vi "RTS Wago Data 4.vi"(8 "Error In":errorcluster, 10 "Station":u8, 11 "Chamber 1 Data in":T1 {"Room PID Settings"."Room Dehumid Temperature I (*RM Dehum I1)" max=30000 step=1; "Room PID Settings"."Room Dehumid Temperature P (*RM Dehum P1)" max=30000 step=1; "Room PID Settings"."Room Cool Temperature I (*RM Cool I1)" max=30000 step=1; "Room PID Settings"."Room Cool Temperature P (*RM Cool P1)" max=30000 step=1; "Room PID Settings"."Room Heat I (*RM Heat I1)" max=30000 step=1; "Room PID Settings"."Room Heat P (*RM Heat P1)" max=30000 step=1; "Room PID Settings"."Room Humidity I (*RM Hum I1)" max=30000 step=1; "Room PID Settings"."Room Humidity P (*RM Hum P1)" max=30000 step=1; "Room PID Settings"."Room Dry I (*RM Dry I1)" max=30000 step=1; "Room PID Settings"."Room Dry P(*RM Dry P1)" max=30000 step=1; "Station 8"."Voltage (V):Element 1 Avg" format="%.3g"; "Station 8"."Voltage (V):Element 2 Avg" format="%.3g"; "Station 8"."Max Watt Hours" format="%.3g"; "Station 8"."Power Factor:Element 2" format="%.3g"; "Station 8"."Power Factor:Element 1" format="%.3g"; "Station 8"."Apparent Power (VA):Element 2" format="%.3g"; "Station 8"."Apparent Power (VA):Element 1" format="%.3g"; "Station 8"."Frequency (Hz):Element 1" format="%.3g"; "Station 8"."Time:Element 1" format="%.3g"; "Station 8"."Voltage Crest Factor:Element 2" format="%.3g"; "Station 8"."Voltage Crest Factor:Element 1" format="%.3g"; "Station 8"."Voltage Harmonic (%):Element 2" format="%.3g"; "Station 8"."Voltage Harmonic (%):Element 1" format="%.3g"; "Station 8"."Current Crest Factor:Element 2" format="%.3g"; "Station 8"."Current Crest Factor:Element 1" format="%.3g"; "Station 8"."Voltage (V):Element 1" format="%.3g"; "Station 8"."Voltage (V):Element 2" format="%.3g"; "Station 8"."Watt Hours (Wh):Sigma" format="%.3f"; "Station 8"."Power (W):Sigma" format="%.3g"; "Station 8"."Current (A):Element 2" format="%.3g"; "Station 8"."Current (A):Element 1" format="%.3g"; "Station 7"."Voltage (V):Element 1 Avg" format="%.3g"; "Station 7"."Voltage (V):Element 2 Avg" format="%.3g"; "Station 7"."Max Watt Hours" format="%.3g"; "Station 7"."Power Factor:Element 2" format="%.3g"; "Station 7"."Power Factor:Element 1" format="%.3g"; "Station 7"."Apparent Power (VA):Element 2" format="%.3g"; "Station 7"."Apparent Power (VA):Element 1" format="%.3g"; "Station 7"."Frequency (Hz):Element 1" format="%.3g"; "Station 7"."Time:Element 1" format="%.3g"; "Station 7"."Voltage Crest Factor:Element 2" format="%.3g"; "Station 7"."Voltage Crest Factor:Element 1" format="%.3g"; "Station 7"."Voltage Harmonic (%):Element 2" format="%.3g"; "Station 7"."Voltage Harmonic (%):Element 1" format="%.3g"; "Station 7"."Current Crest Factor:Element 2" format="%.3g"; "Station 7"."Current Crest Factor:Element 1" format="%.3g"; "Station 7"."Voltage (V):Element 1" format="%.3g"; "Station 7"."Voltage (V):Element 2" format="%.3g"; "Station 7"."Watt Hours (Wh):Sigma" format="%.3f"; "Station 7"."Power (W):Sigma" format="%.3g"; "Station 7"."Current (A):Element 2" format="%.3g"; "Station 7"."Current (A):Element 1" format="%.3g"; "Station 6"."Voltage (V):Element 1 Avg" format="%.3g"; "Station 6"."Voltage (V):Element 2 Avg" format="%.3g"; "Station 6"."Max Watt Hours" format="%.3g"; "Station 6"."Power Factor:Element 2" format="%.3g"; "Station 6"."Power Factor:Element 1" format="%.3g"; "Station 6"."Apparent Power (VA):Element 2" format="%.3g"; "Station 6"."Apparent Power (VA):Element 1" format="%.3g"; "Station 6"."Frequency (Hz):Element 1" format="%.3g"; "Station 6"."Time:Element 1" format="%.3g"; "Station 6"."Voltage Crest Factor:Element 2" format="%.3g"; "Station 6"."Voltage Crest Factor:Element 1" format="%.3g"; "Station 6"."Voltage Harmonic (%):Element 2" format="%.3g"; "Station 6"."Voltage Harmonic (%):Element 1" format="%.3g"; "Station 6"."Current Crest Factor:Element 2" format="%.3g"; "Station 6"."Current Crest Factor:Element 1" format="%.3g"; "Station 6"."Voltage (V):Element 1" format="%.3g"; "Station 6"."Voltage (V):Element 2" format="%.3g"; "Station 6"."Watt Hours (Wh):Sigma" format="%.3f"; "Station 6"."Power (W):Sigma" format="%.3g"; "Station 6"."Current (A):Element 2" format="%.3g"; "Station 6"."Current (A):Element 1" format="%.3g"; "Station 5"."Voltage (V):Element 1 Avg" format="%.3g"; "Station 5"."Voltage (V):Element 2 Avg" format="%.3g"; "Station 5"."Max Watt Hours" format="%.3g"; "Station 5"."Power Factor:Element 2" format="%.3g"; "Station 5"."Power Factor:Element 1" format="%.3g"; "Station 5"."Apparent Power (VA):Element 2" format="%.3g"; "Station 5"."Apparent Power (VA):Element 1" format="%.3g"; "Station 5"."Frequency (Hz):Element 1" format="%.3g"; "Station 5"."Time:Element 1" format="%.3g"; "Station 5"."Voltage Crest Factor:Element 2" format="%.3g"; "Station 5"."Voltage Crest Factor:Element 1" format="%.3g"; "Station 5"."Voltage Harmonic (%):Element 2" format="%.3g"; "Station 5"."Voltage Harmonic (%):Element 1" format="%.3g"; "Station 5"."Current Crest Factor:Element 2" format="%.3g"; "Station 5"."Current Crest Factor:Element 1" format="%.3g"; "Station 5"."Voltage (V):Element 1" format="%.3g"; "Station 5"."Voltage (V):Element 2" format="%.3g"; "Station 5"."Watt Hours (Wh):Sigma" format="%.3f"; "Station 5"."Power (W):Sigma" format="%.3g"; "Station 5"."Current (A):Element 2" format="%.3g"; "Station 5"."Current (A):Element 1" format="%.3g"; "Station 4"."Voltage (V):Element 1 Avg" format="%.3g"; "Station 4"."Voltage (V):Element 2 Avg" format="%.3g"; "Station 4"."Max Watt Hours" format="%.3g"; "Station 4"."Power Factor:Element 2" format="%.3g"; "Station 4"."Power Factor:Element 1" format="%.3g"; "Station 4"."Apparent Power (VA):Element 2" format="%.3g"; "Station 4"."Apparent Power (VA):Element 1" format="%.3g"; "Station 4"."Frequency (Hz):Element 1" format="%.3g"; "Station 4"."Time:Element 1" format="%.3g"; "Station 4"."Voltage Crest Factor:Element 2" format="%.3g"; "Station 4"."Voltage Crest Factor:Element 1" format="%.3g"; "Station 4"."Voltage Harmonic (%):Element 2" format="%.3g"; "Station 4"."Voltage Harmonic (%):Element 1" format="%.3g"; "Station 4"."Current Crest Factor:Element 2" format="%.3g"; "Station 4"."Current Crest Factor:Element 1" format="%.3g"; "Station 4"."Voltage (V):Element 1" format="%.3g"; "Station 4"."Voltage (V):Element 2" format="%.3g"; "Station 4"."Watt Hours (Wh):Sigma" format="%.3f"; "Station 4"."Power (W):Sigma" format="%.3g"; "Station 4"."Current (A):Element 2" format="%.3g"; "Station 4"."Current (A):Element 1" format="%.3g"; "Station 3"."Voltage (V):Element 1 Avg" format="%.3g"; "Station 3"."Voltage (V):Element 2 Avg" format="%.3g"; "Station 3"."Max Watt Hours" format="%.3g"; "Station 3"."Power Factor:Element 2" format="%.3g"; "Station 3"."Power Factor:Element 1" format="%.3g"; "Station 3"."Apparent Power (VA):Element 2" format="%.3g"; "Station 3"."Apparent Power (VA):Element 1" format="%.3g"; "Station 3"."Frequency (Hz):Element 1" format="%.3g"; "Station 3"."Time:Element 1" format="%.3g"; "Station 3"."Voltage Crest Factor:Element 2" format="%.3g"; "Station 3"."Voltage Crest Factor:Element 1" format="%.3g"; "Station 3"."Voltage Harmonic (%):Element 2" format="%.3g"; "Station 3"."Voltage Harmonic (%):Element 1" format="%.3g"; "Station 3"."Current Crest Factor:Element 2" format="%.3g"; "Station 3"."Current Crest Factor:Element 1" format="%.3g"; "Station 3"."Voltage (V):Element 1" format="%.3g"; "Station 3"."Voltage (V):Element 2" format="%.3g"; "Station 3"."Watt Hours (Wh):Sigma" format="%.3f"; "Station 3"."Power (W):Sigma" format="%.3g"; "Station 3"."Current (A):Element 2" format="%.3g"; "Station 3"."Current (A):Element 1" format="%.3g"; "Station 2"."Voltage (V):Element 1 Avg" format="%.3g"; "Station 2"."Voltage (V):Element 2 Avg" format="%.3g"; "Station 2"."Max Watt Hours" format="%.3g"; "Station 2"."Power Factor:Element 2" format="%.3g"; "Station 2"."Power Factor:Element 1" format="%.3g"; "Station 2"."Apparent Power (VA):Element 2" format="%.3g"; "Station 2"."Apparent Power (VA):Element 1" format="%.3g"; "Station 2"."Frequency (Hz):Element 1" format="%.3g"; "Station 2"."Time:Element 1" format="%.3g"; "Station 2"."Voltage Crest Factor:Element 2" format="%.3g"; "Station 2"."Voltage Crest Factor:Element 1" format="%.3g"; "Station 2"."Voltage Harmonic (%):Element 2" format="%.3g"; "Station 2"."Voltage Harmonic (%):Element 1" format="%.3g"; "Station 2"."Current Crest Factor:Element 2" format="%.3g"; "Station 2"."Current Crest Factor:Element 1" format="%.3g"; "Station 2"."Voltage (V):Element 1" format="%.3g"; "Station 2"."Voltage (V):Element 2" format="%.3g"; "Station 2"."Watt Hours (Wh):Sigma" format="%.3f"; "Station 2"."Power (W):Sigma" format="%.3g"; "Station 2"."Current (A):Element 2" format="%.3g"; "Station 2"."Current (A):Element 1" format="%.3g"; "Station 1"."Voltage (V):Element 1 Avg" format="%.3g"; "Station 1"."Voltage (V):Element 2 Avg" format="%.3g"; "Station 1"."Max Watt Hours" format="%.3g"; "Station 1"."Power Factor:Element 2" format="%.3g"; "Station 1"."Power Factor:Element 1" format="%.3g"; "Station 1"."Apparent Power (VA):Element 2" format="%.3g"; "Station 1"."Apparent Power (VA):Element 1" format="%.3g"; "Station 1"."Frequency (Hz):Element 1" format="%.3g"; "Station 1"."Time:Element 1" format="%.3g"; "Station 1"."Voltage Crest Factor:Element 2" format="%.3g"; "Station 1"."Voltage Crest Factor:Element 1" format="%.3g"; "Station 1"."Voltage Harmonic (%):Element 2" format="%.3g"; "Station 1"."Voltage Harmonic (%):Element 1" format="%.3g"; "Station 1"."Current Crest Factor:Element 2" format="%.3g"; "Station 1"."Current Crest Factor:Element 1" format="%.3g"; "Station 1"."Voltage (V):Element 1" format="%.3g"; "Station 1"."Voltage (V):Element 2" format="%.3g"; "Station 1"."Watt Hours (Wh):Sigma" format="%.3f"; "Station 1"."Power (W):Sigma" format="%.3g"; "Station 1"."Current (A):Element 2" format="%.3g"; "Station 1"."Current (A):Element 1" format="%.3g"}) -> (0 "Error Out":errorcluster, 1 "Data 4 (DBL)":dbl[](array[numeric]), 2 "Data 4":string[][](array[string]), 3 "Chamber 1 Data Out":T1 {"Room PID Settings"."Room Dehumid Temperature I (*RM Dehum I1)" max=30000 step=1; "Room PID Settings"."Room Dehumid Temperature P (*RM Dehum P1)" max=30000 step=1; "Room PID Settings"."Room Cool Temperature I (*RM Cool I1)" max=30000 step=1; "Room PID Settings"."Room Cool Temperature P (*RM Cool P1)" max=30000 step=1; "Room PID Settings"."Room Heat I (*RM Heat I1)" max=30000 step=1; "Room PID Settings"."Room Heat P (*RM Heat P1)" max=30000 step=1; "Room PID Settings"."Room Humidity I (*RM Hum I1)" max=30000 step=1; "Room PID Settings"."Room Humidity P (*RM Hum P1)" max=30000 step=1; "Room PID Settings"."Room Dry I (*RM Dry I1)" max=30000 step=1; "Room PID Settings"."Room Dry P(*RM Dry P1)" max=30000 step=1; "Station 8"."Voltage (V):Element 1 Avg" format="%.3g"; "Station 8"."Voltage (V):Element 2 Avg" format="%.3g"; "Station 8"."Max Watt Hours" format="%.3g"; "Station 8"."Power Factor:Element 2" format="%.3g"; "Station 8"."Power Factor:Element 1" format="%.3g"; "Station 8"."Apparent Power (VA):Element 2" format="%.3g"; "Station 8"."Apparent Power (VA):Element 1" format="%.3g"; "Station 8"."Frequency (Hz):Element 1" format="%.3g"; "Station 8"."Time:Element 1" format="%.3g"; "Station 8"."Voltage Crest Factor:Element 2" format="%.3g"; "Station 8"."Voltage Crest Factor:Element 1" format="%.3g"; "Station 8"."Voltage Harmonic (%):Element 2" format="%.3g"; "Station 8"."Voltage Harmonic (%):Element 1" format="%.3g"; "Station 8"."Current Crest Factor:Element 2" format="%.3g"; "Station 8"."Current Crest Factor:Element 1" format="%.3g"; "Station 8"."Voltage (V):Element 1" format="%.3g"; "Station 8"."Voltage (V):Element 2" format="%.3g"; "Station 8"."Watt Hours (Wh):Sigma" format="%.3f"; "Station 8"."Power (W):Sigma" format="%.3g"; "Station 8"."Current (A):Element 2" format="%.3g"; "Station 8"."Current (A):Element 1" format="%.3g"; "Station 7"."Voltage (V):Element 1 Avg" format="%.3g"; "Station 7"."Voltage (V):Element 2 Avg" format="%.3g"; "Station 7"."Max Watt Hours" format="%.3g"; "Station 7"."Power Factor:Element 2" format="%.3g"; "Station 7"."Power Factor:Element 1" format="%.3g"; "Station 7"."Apparent Power (VA):Element 2" format="%.3g"; "Station 7"."Apparent Power (VA):Element 1" format="%.3g"; "Station 7"."Frequency (Hz):Element 1" format="%.3g"; "Station 7"."Time:Element 1" format="%.3g"; "Station 7"."Voltage Crest Factor:Element 2" format="%.3g"; "Station 7"."Voltage Crest Factor:Element 1" format="%.3g"; "Station 7"."Voltage Harmonic (%):Element 2" format="%.3g"; "Station 7"."Voltage Harmonic (%):Element 1" format="%.3g"; "Station 7"."Current Crest Factor:Element 2" format="%.3g"; "Station 7"."Current Crest Factor:Element 1" format="%.3g"; "Station 7"."Voltage (V):Element 1" format="%.3g"; "Station 7"."Voltage (V):Element 2" format="%.3g"; "Station 7"."Watt Hours (Wh):Sigma" format="%.3f"; "Station 7"."Power (W):Sigma" format="%.3g"; "Station 7"."Current (A):Element 2" format="%.3g"; "Station 7"."Current (A):Element 1" format="%.3g"; "Station 6"."Voltage (V):Element 1 Avg" format="%.3g"; "Station 6"."Voltage (V):Element 2 Avg" format="%.3g"; "Station 6"."Max Watt Hours" format="%.3g"; "Station 6"."Power Factor:Element 2" format="%.3g"; "Station 6"."Power Factor:Element 1" format="%.3g"; "Station 6"."Apparent Power (VA):Element 2" format="%.3g"; "Station 6"."Apparent Power (VA):Element 1" format="%.3g"; "Station 6"."Frequency (Hz):Element 1" format="%.3g"; "Station 6"."Time:Element 1" format="%.3g"; "Station 6"."Voltage Crest Factor:Element 2" format="%.3g"; "Station 6"."Voltage Crest Factor:Element 1" format="%.3g"; "Station 6"."Voltage Harmonic (%):Element 2" format="%.3g"; "Station 6"."Voltage Harmonic (%):Element 1" format="%.3g"; "Station 6"."Current Crest Factor:Element 2" format="%.3g"; "Station 6"."Current Crest Factor:Element 1" format="%.3g"; "Station 6"."Voltage (V):Element 1" format="%.3g"; "Station 6"."Voltage (V):Element 2" format="%.3g"; "Station 6"."Watt Hours (Wh):Sigma" format="%.3f"; "Station 6"."Power (W):Sigma" format="%.3g"; "Station 6"."Current (A):Element 2" format="%.3g"; "Station 6"."Current (A):Element 1" format="%.3g"; "Station 5"."Voltage (V):Element 1 Avg" format="%.3g"; "Station 5"."Voltage (V):Element 2 Avg" format="%.3g"; "Station 5"."Max Watt Hours" format="%.3g"; "Station 5"."Power Factor:Element 2" format="%.3g"; "Station 5"."Power Factor:Element 1" format="%.3g"; "Station 5"."Apparent Power (VA):Element 2" format="%.3g"; "Station 5"."Apparent Power (VA):Element 1" format="%.3g"; "Station 5"."Frequency (Hz):Element 1" format="%.3g"; "Station 5"."Time:Element 1" format="%.3g"; "Station 5"."Voltage Crest Factor:Element 2" format="%.3g"; "Station 5"."Voltage Crest Factor:Element 1" format="%.3g"; "Station 5"."Voltage Harmonic (%):Element 2" format="%.3g"; "Station 5"."Voltage Harmonic (%):Element 1" format="%.3g"; "Station 5"."Current Crest Factor:Element 2" format="%.3g"; "Station 5"."Current Crest Factor:Element 1" format="%.3g"; "Station 5"."Voltage (V):Element 1" format="%.3g"; "Station 5"."Voltage (V):Element 2" format="%.3g"; "Station 5"."Watt Hours (Wh):Sigma" format="%.3f"; "Station 5"."Power (W):Sigma" format="%.3g"; "Station 5"."Current (A):Element 2" format="%.3g"; "Station 5"."Current (A):Element 1" format="%.3g"; "Station 4"."Voltage (V):Element 1 Avg" format="%.3g"; "Station 4"."Voltage (V):Element 2 Avg" format="%.3g"; "Station 4"."Max Watt Hours" format="%.3g"; "Station 4"."Power Factor:Element 2" format="%.3g"; "Station 4"."Power Factor:Element 1" format="%.3g"; "Station 4"."Apparent Power (VA):Element 2" format="%.3g"; "Station 4"."Apparent Power (VA):Element 1" format="%.3g"; "Station 4"."Frequency (Hz):Element 1" format="%.3g"; "Station 4"."Time:Element 1" format="%.3g"; "Station 4"."Voltage Crest Factor:Element 2" format="%.3g"; "Station 4"."Voltage Crest Factor:Element 1" format="%.3g"; "Station 4"."Voltage Harmonic (%):Element 2" format="%.3g"; "Station 4"."Voltage Harmonic (%):Element 1" format="%.3g"; "Station 4"."Current Crest Factor:Element 2" format="%.3g"; "Station 4"."Current Crest Factor:Element 1" format="%.3g"; "Station 4"."Voltage (V):Element 1" format="%.3g"; "Station 4"."Voltage (V):Element 2" format="%.3g"; "Station 4"."Watt Hours (Wh):Sigma" format="%.3f"; "Station 4"."Power (W):Sigma" format="%.3g"; "Station 4"."Current (A):Element 2" format="%.3g"; "Station 4"."Current (A):Element 1" format="%.3g"; "Station 3"."Voltage (V):Element 1 Avg" format="%.3g"; "Station 3"."Voltage (V):Element 2 Avg" format="%.3g"; "Station 3"."Max Watt Hours" format="%.3g"; "Station 3"."Power Factor:Element 2" format="%.3g"; "Station 3"."Power Factor:Element 1" format="%.3g"; "Station 3"."Apparent Power (VA):Element 2" format="%.3g"; "Station 3"."Apparent Power (VA):Element 1" format="%.3g"; "Station 3"."Frequency (Hz):Element 1" format="%.3g"; "Station 3"."Time:Element 1" format="%.3g"; "Station 3"."Voltage Crest Factor:Element 2" format="%.3g"; "Station 3"."Voltage Crest Factor:Element 1" format="%.3g"; "Station 3"."Voltage Harmonic (%):Element 2" format="%.3g"; "Station 3"."Voltage Harmonic (%):Element 1" format="%.3g"; "Station 3"."Current Crest Factor:Element 2" format="%.3g"; "Station 3"."Current Crest Factor:Element 1" format="%.3g"; "Station 3"."Voltage (V):Element 1" format="%.3g"; "Station 3"."Voltage (V):Element 2" format="%.3g"; "Station 3"."Watt Hours (Wh):Sigma" format="%.3f"; "Station 3"."Power (W):Sigma" format="%.3g"; "Station 3"."Current (A):Element 2" format="%.3g"; "Station 3"."Current (A):Element 1" format="%.3g"; "Station 2"."Voltage (V):Element 1 Avg" format="%.3g"; "Station 2"."Voltage (V):Element 2 Avg" format="%.3g"; "Station 2"."Max Watt Hours" format="%.3g"; "Station 2"."Power Factor:Element 2" format="%.3g"; "Station 2"."Power Factor:Element 1" format="%.3g"; "Station 2"."Apparent Power (VA):Element 2" format="%.3g"; "Station 2"."Apparent Power (VA):Element 1" format="%.3g"; "Station 2"."Frequency (Hz):Element 1" format="%.3g"; "Station 2"."Time:Element 1" format="%.3g"; "Station 2"."Voltage Crest Factor:Element 2" format="%.3g"; "Station 2"."Voltage Crest Factor:Element 1" format="%.3g"; "Station 2"."Voltage Harmonic (%):Element 2" format="%.3g"; "Station 2"."Voltage Harmonic (%):Element 1" format="%.3g"; "Station 2"."Current Crest Factor:Element 2" format="%.3g"; "Station 2"."Current Crest Factor:Element 1" format="%.3g"; "Station 2"."Voltage (V):Element 1" format="%.3g"; "Station 2"."Voltage (V):Element 2" format="%.3g"; "Station 2"."Watt Hours (Wh):Sigma" format="%.3f"; "Station 2"."Power (W):Sigma" format="%.3g"; "Station 2"."Current (A):Element 2" format="%.3g"; "Station 2"."Current (A):Element 1" format="%.3g"; "Station 1"."Voltage (V):Element 1 Avg" format="%.3g"; "Station 1"."Voltage (V):Element 2 Avg" format="%.3g"; "Station 1"."Max Watt Hours" format="%.3g"; "Station 1"."Power Factor:Element 2" format="%.3g"; "Station 1"."Power Factor:Element 1" format="%.3g"; "Station 1"."Apparent Power (VA):Element 2" format="%.3g"; "Station 1"."Apparent Power (VA):Element 1" format="%.3g"; "Station 1"."Frequency (Hz):Element 1" format="%.3g"; "Station 1"."Time:Element 1" format="%.3g"; "Station 1"."Voltage Crest Factor:Element 2" format="%.3g"; "Station 1"."Voltage Crest Factor:Element 1" format="%.3g"; "Station 1"."Voltage Harmonic (%):Element 2" format="%.3g"; "Station 1"."Voltage Harmonic (%):Element 1" format="%.3g"; "Station 1"."Current Crest Factor:Element 2" format="%.3g"; "Station 1"."Current Crest Factor:Element 1" format="%.3g"; "Station 1"."Voltage (V):Element 1" format="%.3g"; "Station 1"."Voltage (V):Element 2" format="%.3g"; "Station 1"."Watt Hours (Wh):Sigma" format="%.3f"; "Station 1"."Power (W):Sigma" format="%.3g"; "Station 1"."Current (A):Element 2" format="%.3g"; "Station 1"."Current (A):Element 1" format="%.3g"})   [LabVIEW 2016]
uses:
  Type Definitions/RTS Chamber Data.ctl
  Utility/Type Definitions/UTILITY Power Data.ctl
  Type Definitions/RTS Chamber TCs.ctl
  Type Definitions/RTS MX5 AUX Data.ctl
  Drivers/WAGO 750-881/Type Definitions/Wago Door Relays.ctl
  Drivers/WAGO 750-881/Type Definitions/Wago Contactor Settings.ctl
  Drivers/WAGO 750-881/Type Definitions/Wago Ground Leakage.ctl
  Drivers/WAGO 750-881/Type Definitions/Wago Measured Input Data.ctl
  Drivers/WAGO 750-881/Type Definitions/Wago Room Setpoint Targets.ctl
  Drivers/WAGO 750-881/Type Definitions/Wago Room PID Settings.ctl
  Drivers/WAGO 750-881/Type Definitions/Wago Room Condtions.ctl
panel:
  # "APLUS"
  # "MX100"
  # "Wago Controller"
  # "APLUS"
  # "MX100"
  # "Wago Controller"
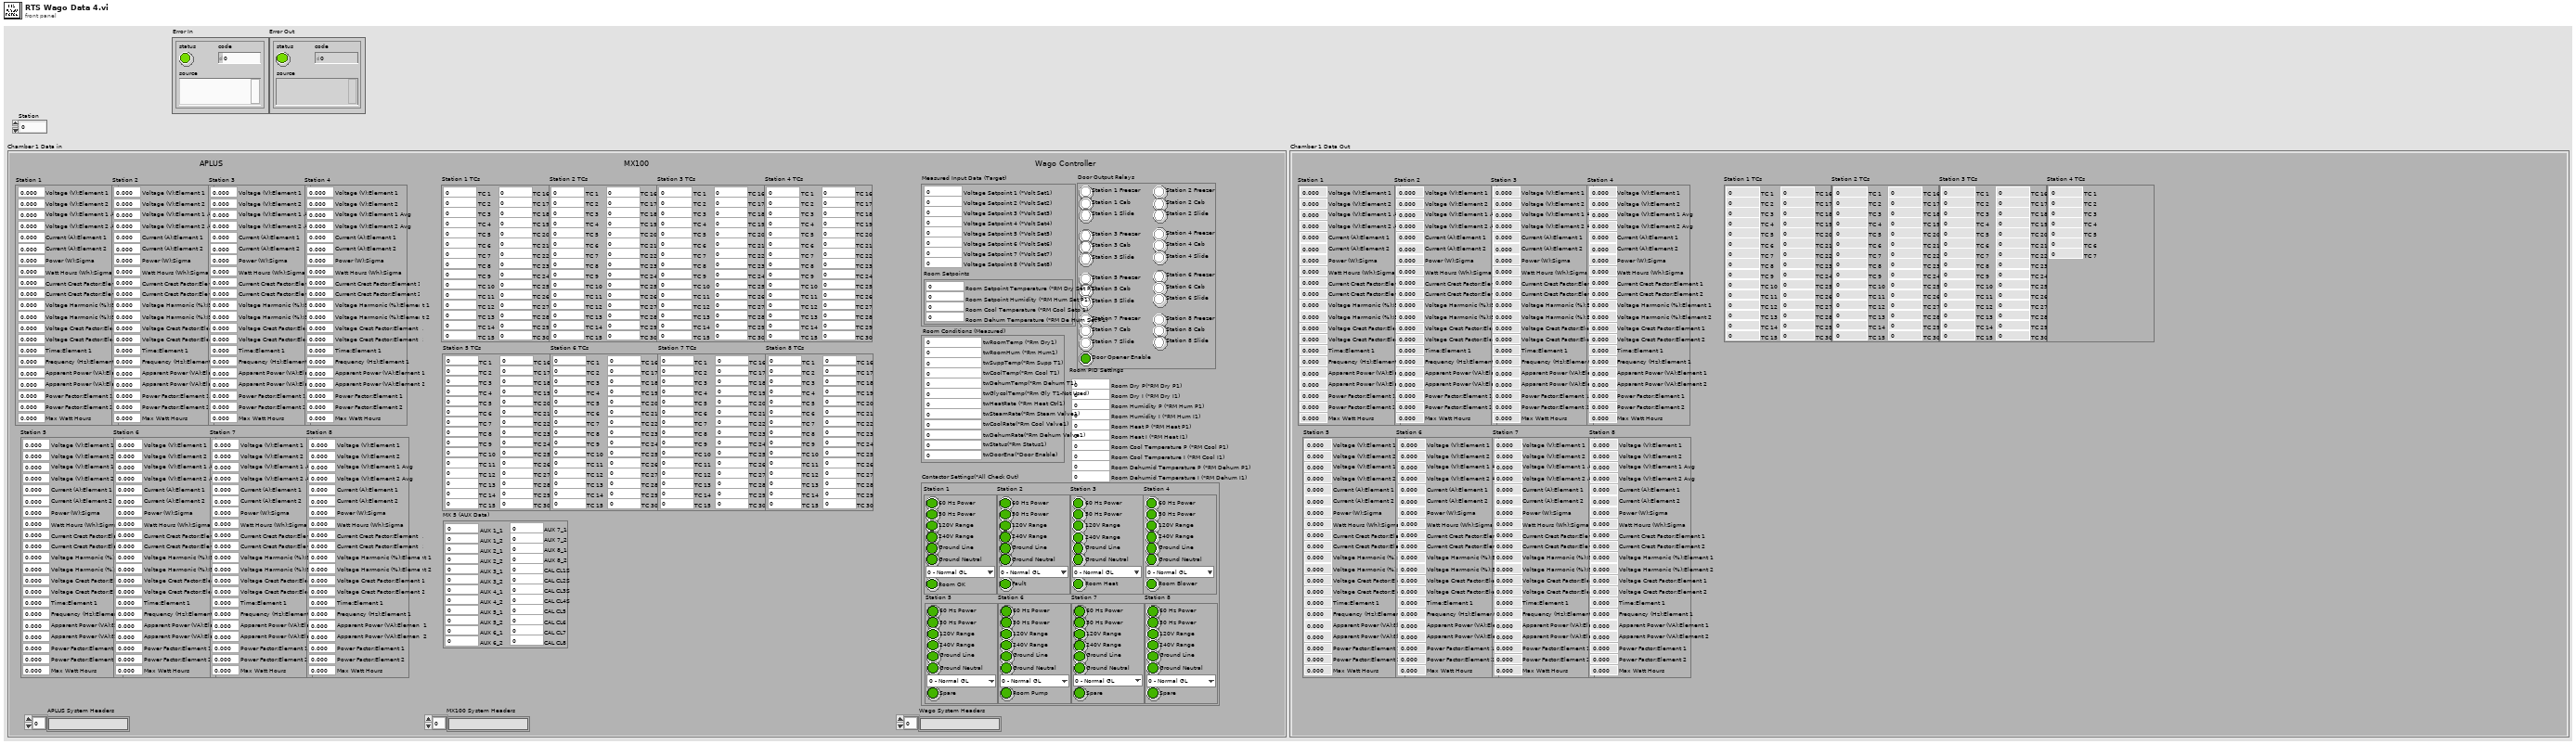
[diagram p1: front panel]
types:
  T1 = typedef "RTS Chamber Data.ctl" = cluster{"Station 1":T2, "Station 2":T2, "Station 3":T2, "Station 4":T2, "Station 5":T2, "Station 6":T2, "Station 7":T2, "Station 8":T2, "Station 1 TCs":T3, "Station 2 TCs":T3, "Station 3 TCs":T3, "Station 4 TCs":T3, "Station 5 TCs":T3, "Station 6 TCs":T3, "Station 7 TCs":T3, "Station 8 TCs":T3, "MX 5 (AUX Data)":T4, "Door Output Relays":T5, "Contactor Settings(*All Check Out)":T6, "Measured Input Data (Target)":T8, "Room PID Settings":T10, "Room Conditions (Measured)":T11, "APLUS System Headers":string[], "MX100 System Headers":string[], "Wago System Headers":string[]}
  T2 = typedef "UTILITY Power Data.ctl" = cluster{"Current (A):Element 1":dbl, "Current (A):Element 2":dbl, "Power (W):Sigma":dbl, "Watt Hours (Wh):Sigma":dbl, "Voltage (V):Element 2":dbl, "Voltage (V):Element 1":dbl, "Current Crest Factor:Element 1":dbl, "Current Crest Factor:Element 2":dbl, "Voltage Harmonic (%):Element 1":dbl, "Voltage Harmonic (%):Element 2":dbl, "Voltage Crest Factor:Element 1":dbl, "Voltage Crest Factor:Element 2":dbl, "Time:Element 1":dbl, "Frequency (Hz):Element 1":dbl, "Apparent Power (VA):Element 1":dbl, "Apparent Power (VA):Element 2":dbl, "Power Factor:Element 1":dbl, "Power Factor:Element 2":dbl, "Max Watt Hours":dbl, "Voltage (V):Element 2 Avg":dbl, "Voltage (V):Element 1 Avg":dbl}
  T3 = typedef "RTS Chamber TCs.ctl" = cluster{"TC 1":dbl, "TC 2":dbl, "TC 3":dbl, "TC 4":dbl, "TC 5":dbl, "TC 6":dbl, "TC 7":dbl, "TC 8":dbl, "TC 9":dbl, "TC 10":dbl, "TC 11":dbl, "TC 12":dbl, "TC 13":dbl, "TC 14":dbl, "TC 15":dbl, "TC 16":dbl, "TC 17":dbl, "TC 18":dbl, "TC 19":dbl, "TC 20":dbl, "TC 21":dbl, "TC 22":dbl, "TC 23":dbl, "TC 24":dbl, "TC 25":dbl, "TC 26":dbl, "TC 27":dbl, "TC 28":dbl, "TC 29":dbl, "TC 30":dbl}
  T4 = typedef "RTS MX5 AUX Data.ctl" = cluster{"AUX 1_1":dbl, "AUX 1_2":dbl, "AUX 2_1":dbl, "AUX 2_2":dbl, "AUX 3_1":dbl, "AUX 3_2":dbl, "AUX 4_1":dbl, "AUX 4_2":dbl, "AUX 5_1":dbl, "AUX 5_2":dbl, "AUX 6_1":dbl, "AUX 6_2":dbl, "AUX 7_1":dbl, "AUX 7_2":dbl, "AUX 8_1":dbl, "AUX 8_2":dbl, "CAL CL1S":dbl, "CAL CL2S":dbl, "CAL CL3S":dbl, "CAL CL4S":dbl, "CAL CL5":dbl, "CAL CL6":dbl, "CAL CL7":dbl, "CAL CL8":dbl}
  T5 = typedef "Wago Door Relays.ctl" = cluster{"Station 1 Freezer":bool, "Station 1 Cab":bool, "Station 1 Slide":bool, "Station 2 Freezer":bool, "Station 2 Cab":bool, "Station 2 Slide":bool, "Station 3 Freezer":bool, "Station 3 Cab":bool, "Station 3 Slide":bool, "Station 4 Freezer":bool, "Station 4 Cab":bool, "Station 4 Slide":bool, "Station 5 Freezer":bool, "Station 5 Cab":bool, "Station 5 Slide":bool, "Station 6 Freezer":bool, "Station 6 Cab":bool, "Station 6 Slide":bool, "Station 7 Freezer":bool, "Station 7 Cab":bool, "Station 7 Slide":bool, "Station 8 Freezer":bool, "Station 8 Cab":bool, "Station 8 Slide":bool, "Door Opener Enable":bool}
  T6 = typedef "Wago Contactor Settings.ctl" = cluster{"Station 1":cluster{"60 Hz Power":bool, "50 Hz Power":bool, "120V Range":bool, "240V Range":bool, "Ground Line":bool, "Ground Neutral":bool, "Room OK":bool, "Ground Leakage":T7}, "Station 2":cluster{"60 Hz Power":bool, "50 Hz Power":bool, "120V Range":bool, "240V Range":bool, "Ground Line":bool, "Ground Neutral":bool, "Fault":bool, "Ground Leakage":T7}, "Station 3":cluster{"60 Hz Power":bool, "50 Hz Power":bool, "120V Range":bool, "240V Range":bool, "Ground Line":bool, "Ground Neutral":bool, "Room Heat":bool, "Ground Leakage":T7}, "Station 4":cluster{"60 Hz Power":bool, "50 Hz Power":bool, "120V Range":bool, "240V Range":bool, "Ground Line":bool, "Ground Neutral":bool, "Room Blower":bool, "Ground Leakage":T7}, "Station 5":cluster{"60 Hz Power":bool, "50 Hz Power":bool, "120V Range":bool, "240V Range":bool, "Ground Line":bool, "Ground Neutral":bool, "Spare":bool, "Ground Leakage":T7}, "Station 6":cluster{"60 Hz Power":bool, "50 Hz Power":bool, "120V Range":bool, "240V Range":bool, "Ground Line":bool, "Ground Neutral":bool, "Room Pump":bool, "Ground Leakage":T7}, "Station 7":cluster{"60 Hz Power":bool, "50 Hz Power":bool, "120V Range":bool, "240V Range":bool, "Ground Line":bool, "Ground Neutral":bool, "Spare":bool, "Ground Leakage":T7}, "Station 8":cluster{"60 Hz Power":bool, "50 Hz Power":bool, "120V Range":bool, "240V Range":bool, "Ground Line":bool, "Ground Neutral":bool, "Spare":bool, "Ground Leakage":T7}}
  T7 = typedef "Wago Ground Leakage.ctl" = enum16{"0 - Normal GL", "1 - Measure GL"}
  T8 = typedef "Wago Measured Input Data.ctl" = cluster{"Voltage Setpoint 1 (*Volt Set1)":dbl, "Voltage Setpoint 2 (*Volt Set2)":dbl, "Voltage Setpoint 3 (*Volt Set3)":dbl, "Voltage Setpoint 4 (*Volt Set4)":dbl, "Voltage Setpoint 5 (*Volt Set5)":dbl, "Voltage Setpoint 6 (*Volt Set6)":dbl, "Voltage Setpoint 7 (*Volt Set7)":dbl, "Voltage Setpoint 8 (*Volt Set8)":dbl, "Room Setpoints":T9}
  T9 = typedef "Wago Room Setpoint Targets.ctl" = cluster{"Room Setpoint Temperature (*RM Dry Set P1)":dbl, "Room Setpoint Humidity (*RM Hum Set P1)":dbl, "Room Cool Temperature (*RM Cool Setp 1)":dbl, "Room Dehum Temperature (*RM De Hum Set P1)":dbl}
  T10 = typedef "Wago Room PID Settings.ctl" = cluster{"Room Dry P(*RM Dry P1)":u16, "Room Dry I (*RM Dry I1)":u16, "Room Humidity P (*RM Hum P1)":u16, "Room Humidity I (*RM Hum I1)":u16, "Room Heat P (*RM Heat P1)":u16, "Room Heat I (*RM Heat I1)":u16, "Room Cool Temperature P (*RM Cool P1)":u16, "Room Cool Temperature I (*RM Cool I1)":u16, "Room Dehumid Temperature P (*RM Dehum P1)":u16, "Room Dehumid Temperature I (*RM Dehum I1)":u16}
  T11 = typedef "Wago Room Condtions.ctl" = cluster{"twDoorEna(*Door Enable)":u16, "twStatus(*Rm Status1)":u16, "twRoomTemp (*Rm Dry1)":dbl, "twRoomHum (*Rm Hum1)":dbl, "twSuppTemp(*Rm Supp T1)":dbl, "twCoolTemp(*Rm Cool T1)":dbl, "twDehumTemp(*Rm Dehum T1)":dbl, "twGlycolTemp(*Rm Gly T1-Not Used)":dbl, "twDehumRate(*Rm Dehum Valve1)":dbl, "twCoolRate(*Rm Cool Valve1)":dbl, "twSteamRate(*Rm Steam Valve1)":dbl, "twHeatRate (*Rm Heat Ctrl1)":dbl}
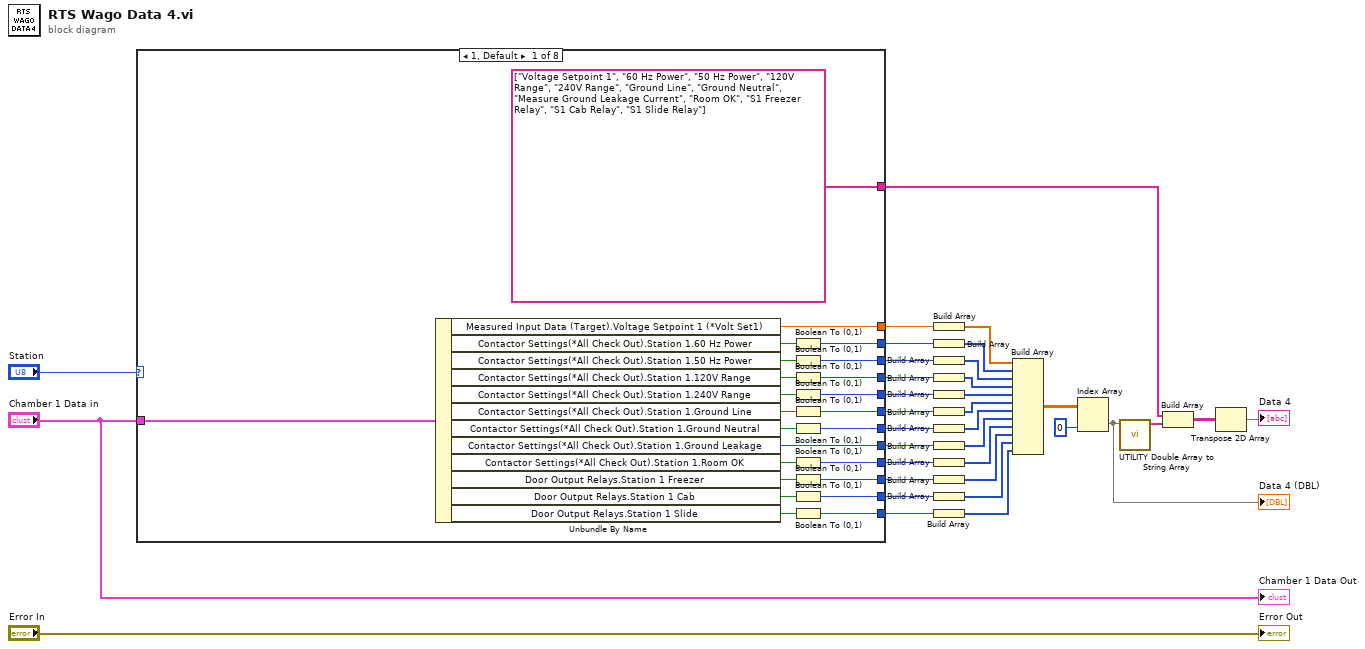
[diagram p0: block diagram]
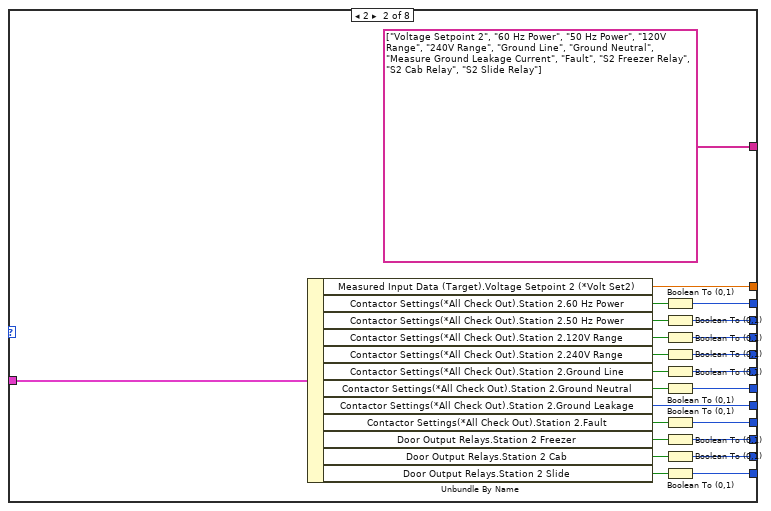
[diagram p2: hidden frame]
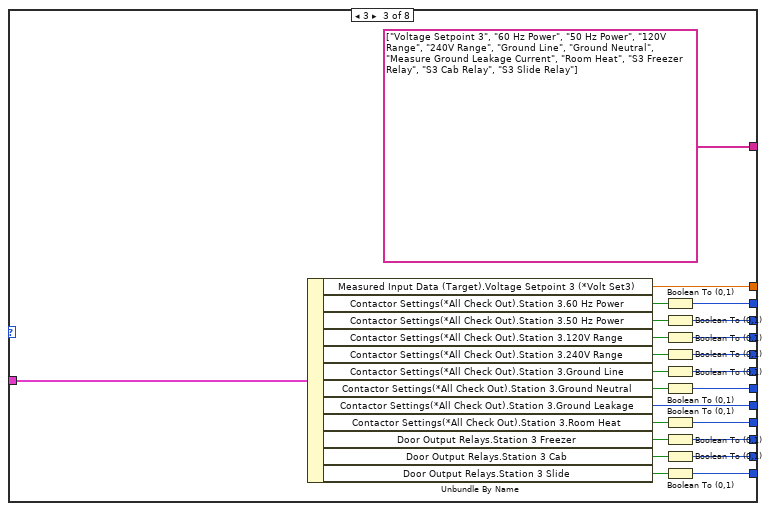
[diagram p3: hidden frame]
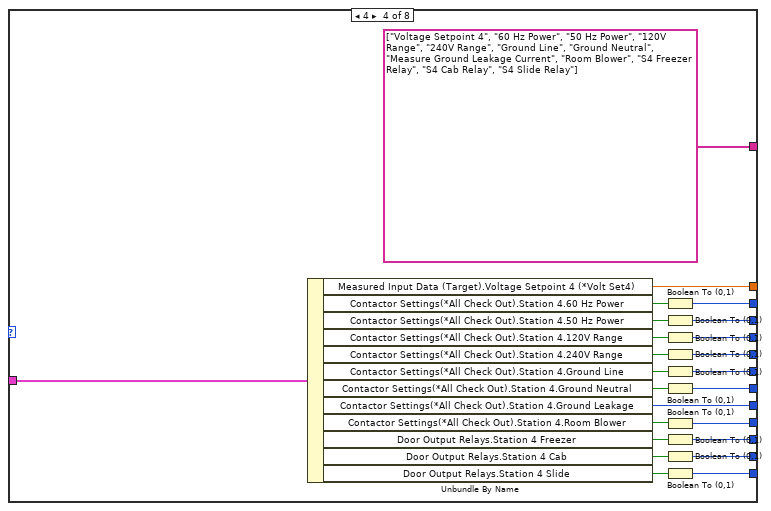
[diagram p4: hidden frame]
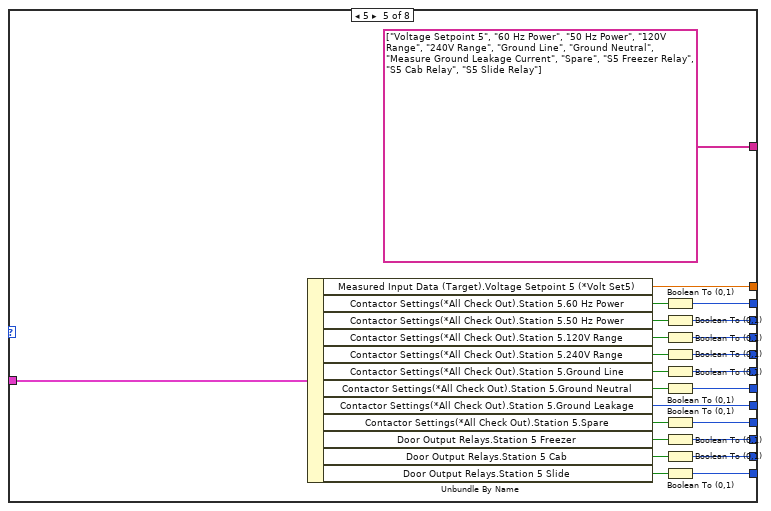
[diagram p5: hidden frame]
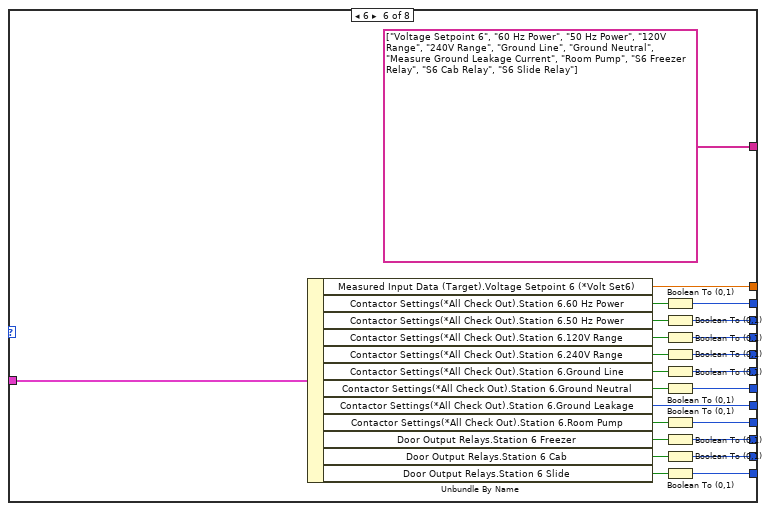
[diagram p6: hidden frame]
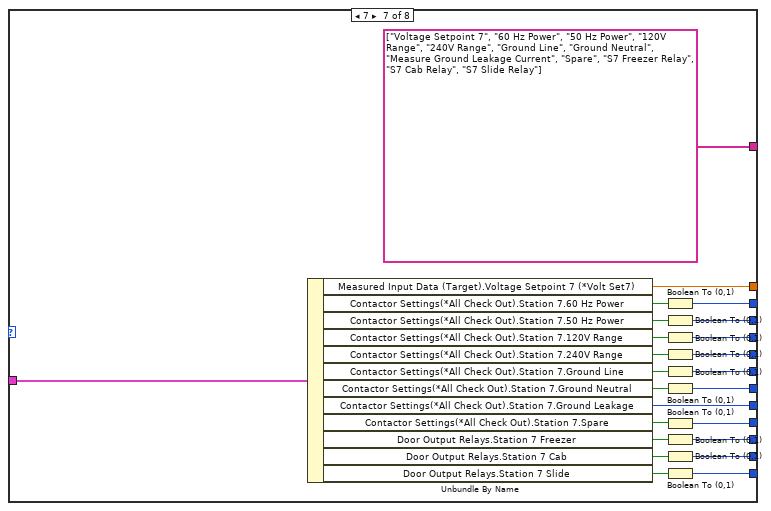
[diagram p7: hidden frame]
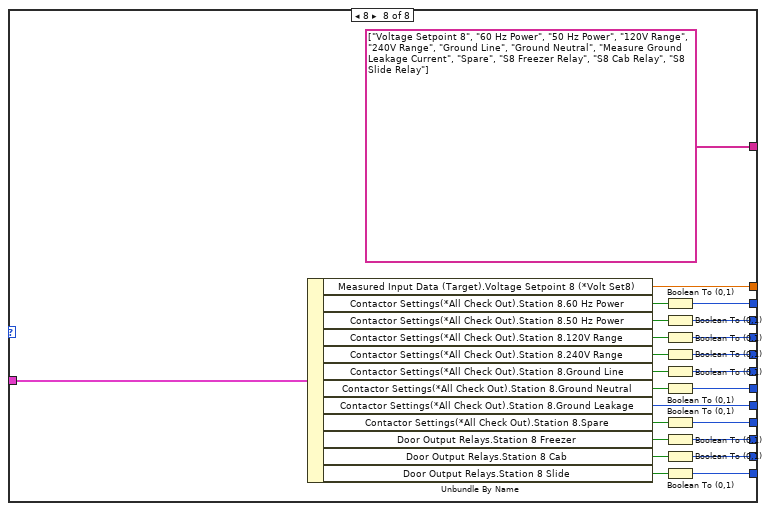
[diagram p8: hidden frame]
diagram:
  n1 = case shown="1, Default" "Station" {
    tunnel: [string[] ["Voltage Setpoint 1", "60 Hz Power", "50 Hz Power", "120V Range", "240V Range", "Ground Line", "Ground Neutral", "Measure Ground Leakage Current", "Room OK", "S1 Freezer Relay", "S1 Cab Relay", "S1 Slide Relay"] string[] ["Voltage Setpoint 2", "60 Hz Power", "50 Hz Power", "120V Range", "240V Range", "Ground Line", "Ground Neutral", "Measure Ground Leakage Current", "Fault", "S2 Freezer Relay", "S2 Cab Relay", "S2 Slide Relay"] string[] ["Voltage Setpoint 3", "60 Hz Power", "50 Hz Power", "120V Range", "240V Range", "Ground Line", "Ground Neutral", "Measure Ground Leakage Current", "Room Heat", "S3 Freezer Relay", "S3 Cab Relay", "S3 Slide Relay"] string[] ["Voltage Setpoint 4", "60 Hz Power", "50 Hz Power", "120V Range", "240V Range", "Ground Line", "Ground Neutral", "Measure Ground Leakage Current", "Room Blower", "S4 Freezer Relay", "S4 Cab Relay", "S4 Slide Relay"] string[] ["Voltage Setpoint 5", "60 Hz Power", "50 Hz Power", "120V Range", "240V Range", "Ground Line", "Ground Neutral", "Measure Ground Leakage Current", "Spare", "S5 Freezer Relay", "S5 Cab Relay", "S5 Slide Relay"] string[] ["Voltage Setpoint 6", "60 Hz Power", "50 Hz Power", "120V Range", "240V Range", "Ground Line", "Ground Neutral", "Measure Ground Leakage Current", "Room Pump", "S6 Freezer Relay", "S6 Cab Relay", "S6 Slide Relay"] string[] ["Voltage Setpoint 7", "60 Hz Power", "50 Hz Power", "120V Range", "240V Range", "Ground Line", "Ground Neutral", "Measure Ground Leakage Current", "Spare", "S7 Freezer Relay", "S7 Cab Relay", "S7 Slide Relay"] string[] ["Voltage Setpoint 8", "60 Hz Power", "50 Hz Power", "120V Range", "240V Range", "Ground Line", "Ground Neutral", "Measure Ground Leakage Current", "Spare", "S8 Freezer Relay", "S8 Cab Relay", "S8 Slide Relay"]] -> w22
    tunnel: [w48 w71 w95 w119 w143 w167 w191 w215] -> w6
    tunnel: [w36 w60 w83 w108 w131 w155 w179 w203] -> w14
    tunnel: [w47 w70 w94 w110 w142 w158 w190 w214] -> w7
    tunnel: [w46 w69 w93 w111 w141 w159 w189 w213] -> w8
    tunnel: [w45 w68 w92 w112 w140 w160 w188 w212] -> w9
    tunnel: [w44 w67 w91 w113 w139 w161 w187 w211] -> w10
    tunnel: [w43 w66 w90 w114 w138 w162 w186 w210] -> w11
    tunnel: [w42 w65 w89 w115 w137 w163 w185 w209] -> w12
    tunnel: [w35 w59 w85 w107 w133 w157 w181 w205] -> w13
    tunnel: [w41 w64 w88 w116 w136 w164 w184 w208] -> w15
    tunnel: [w40 w63 w87 w117 w135 w165 w183 w207] -> w16
    tunnel: [w39 w62 w86 w118 w134 w166 w182 w206] -> w17
    tunnel: "Chamber 1 Data in" -> [w38 w81 w105 w129 w153 w177 w201 w225]
    frame 1, Default {
      n2 = Unbundle By Name(w38) -> ("Measured Input Data (Target).Voltage Setpoint 1 (*Volt Set1)"=w48:dbl, "Contactor Settings(*All Check Out).Station 1.60 Hz Power"=w49:bool, "Contactor Settings(*All Check Out).Station 1.50 Hz Power"=w50:bool, "Contactor Settings(*All Check Out).Station 1.120V Range"=w51:bool, "Contactor Settings(*All Check Out).Station 1.240V Range"=w52:bool, "Contactor Settings(*All Check Out).Station 1.Ground Line"=w53:bool, "Contactor Settings(*All Check Out).Station 1.Ground Neutral"=w54:bool, "Contactor Settings(*All Check Out).Station 1.Ground Leakage"=w35:T7, "Contactor Settings(*All Check Out).Station 1.Room OK"=w37:bool, "Door Output Relays.Station 1 Freezer"=w55:bool, "Door Output Relays.Station 1 Cab"=w56:bool, "Door Output Relays.Station 1 Slide"=w57:bool)
      n3 = Boolean To (0,1)(Boolean=w49) -> (0, 1=w47:i16)
      n4 = Boolean To (0,1)(Boolean=w50) -> (0, 1=w46:i16)
      n5 = Boolean To (0,1)(Boolean=w51) -> (0, 1=w45:i16)
      n6 = Boolean To (0,1)(Boolean=w52) -> (0, 1=w44:i16)
      n7 = Boolean To (0,1)(Boolean=w53) -> (0, 1=w43:i16)
      n8 = Boolean To (0,1)(Boolean=w54) -> (0, 1=w42:i16)
      n9 = Boolean To (0,1)(Boolean=w37) -> (0, 1=w36:i16)
      n10 = Boolean To (0,1)(Boolean=w55) -> (0, 1=w41:i16)
      n11 = Boolean To (0,1)(Boolean=w56) -> (0, 1=w40:i16)
      n12 = Boolean To (0,1)(Boolean=w57) -> (0, 1=w39:i16)
    }
    frame 2 {
      n13 = Unbundle By Name(w81) -> ("Measured Input Data (Target).Voltage Setpoint 2 (*Volt Set2)"=w71:dbl, "Contactor Settings(*All Check Out).Station 2.60 Hz Power"=w72:bool, "Contactor Settings(*All Check Out).Station 2.50 Hz Power"=w73:bool, "Contactor Settings(*All Check Out).Station 2.120V Range"=w74:bool, "Contactor Settings(*All Check Out).Station 2.240V Range"=w75:bool, "Contactor Settings(*All Check Out).Station 2.Ground Line"=w76:bool, "Contactor Settings(*All Check Out).Station 2.Ground Neutral"=w77:bool, "Contactor Settings(*All Check Out).Station 2.Ground Leakage"=w59:T7, "Contactor Settings(*All Check Out).Station 2.Fault"=w61:bool, "Door Output Relays.Station 2 Freezer"=w78:bool, "Door Output Relays.Station 2 Cab"=w79:bool, "Door Output Relays.Station 2 Slide"=w80:bool)
      n14 = Boolean To (0,1)(Boolean=w72) -> (0, 1=w70:i16)
      n15 = Boolean To (0,1)(Boolean=w73) -> (0, 1=w69:i16)
      n16 = Boolean To (0,1)(Boolean=w74) -> (0, 1=w68:i16)
      n17 = Boolean To (0,1)(Boolean=w75) -> (0, 1=w67:i16)
      n18 = Boolean To (0,1)(Boolean=w76) -> (0, 1=w66:i16)
      n19 = Boolean To (0,1)(Boolean=w77) -> (0, 1=w65:i16)
      n20 = Boolean To (0,1)(Boolean=w61) -> (0, 1=w60:i16)
      n21 = Boolean To (0,1)(Boolean=w78) -> (0, 1=w64:i16)
      n22 = Boolean To (0,1)(Boolean=w79) -> (0, 1=w63:i16)
      n23 = Boolean To (0,1)(Boolean=w80) -> (0, 1=w62:i16)
    }
    frame 3 {
      n24 = Unbundle By Name(w105) -> ("Measured Input Data (Target).Voltage Setpoint 3 (*Volt Set3)"=w95:dbl, "Contactor Settings(*All Check Out).Station 3.60 Hz Power"=w96:bool, "Contactor Settings(*All Check Out).Station 3.50 Hz Power"=w97:bool, "Contactor Settings(*All Check Out).Station 3.120V Range"=w98:bool, "Contactor Settings(*All Check Out).Station 3.240V Range"=w99:bool, "Contactor Settings(*All Check Out).Station 3.Ground Line"=w100:bool, "Contactor Settings(*All Check Out).Station 3.Ground Neutral"=w101:bool, "Contactor Settings(*All Check Out).Station 3.Ground Leakage"=w85:T7, "Contactor Settings(*All Check Out).Station 3.Room Heat"=w84:bool, "Door Output Relays.Station 3 Freezer"=w102:bool, "Door Output Relays.Station 3 Cab"=w103:bool, "Door Output Relays.Station 3 Slide"=w104:bool)
      n25 = Boolean To (0,1)(Boolean=w96) -> (0, 1=w94:i16)
      n26 = Boolean To (0,1)(Boolean=w97) -> (0, 1=w93:i16)
      n27 = Boolean To (0,1)(Boolean=w98) -> (0, 1=w92:i16)
      n28 = Boolean To (0,1)(Boolean=w99) -> (0, 1=w91:i16)
      n29 = Boolean To (0,1)(Boolean=w100) -> (0, 1=w90:i16)
      n30 = Boolean To (0,1)(Boolean=w101) -> (0, 1=w89:i16)
      n31 = Boolean To (0,1)(Boolean=w84) -> (0, 1=w83:i16)
      n32 = Boolean To (0,1)(Boolean=w102) -> (0, 1=w88:i16)
      n33 = Boolean To (0,1)(Boolean=w103) -> (0, 1=w87:i16)
      n34 = Boolean To (0,1)(Boolean=w104) -> (0, 1=w86:i16)
    }
    frame 4 {
      n35 = Unbundle By Name(w129) -> ("Measured Input Data (Target).Voltage Setpoint 4 (*Volt Set4)"=w119:dbl, "Contactor Settings(*All Check Out).Station 4.60 Hz Power"=w120:bool, "Contactor Settings(*All Check Out).Station 4.50 Hz Power"=w121:bool, "Contactor Settings(*All Check Out).Station 4.120V Range"=w122:bool, "Contactor Settings(*All Check Out).Station 4.240V Range"=w123:bool, "Contactor Settings(*All Check Out).Station 4.Ground Line"=w124:bool, "Contactor Settings(*All Check Out).Station 4.Ground Neutral"=w125:bool, "Contactor Settings(*All Check Out).Station 4.Ground Leakage"=w107:T7, "Contactor Settings(*All Check Out).Station 4.Room Blower"=w109:bool, "Door Output Relays.Station 4 Freezer"=w126:bool, "Door Output Relays.Station 4 Cab"=w127:bool, "Door Output Relays.Station 4 Slide"=w128:bool)
      n36 = Boolean To (0,1)(Boolean=w120) -> (0, 1=w110:i16)
      n37 = Boolean To (0,1)(Boolean=w121) -> (0, 1=w111:i16)
      n38 = Boolean To (0,1)(Boolean=w122) -> (0, 1=w112:i16)
      n39 = Boolean To (0,1)(Boolean=w123) -> (0, 1=w113:i16)
      n40 = Boolean To (0,1)(Boolean=w124) -> (0, 1=w114:i16)
      n41 = Boolean To (0,1)(Boolean=w125) -> (0, 1=w115:i16)
      n42 = Boolean To (0,1)(Boolean=w109) -> (0, 1=w108:i16)
      n43 = Boolean To (0,1)(Boolean=w126) -> (0, 1=w116:i16)
      n44 = Boolean To (0,1)(Boolean=w127) -> (0, 1=w117:i16)
      n45 = Boolean To (0,1)(Boolean=w128) -> (0, 1=w118:i16)
    }
    frame 5 {
      n46 = Unbundle By Name(w153) -> ("Measured Input Data (Target).Voltage Setpoint 5 (*Volt Set5)"=w143:dbl, "Contactor Settings(*All Check Out).Station 5.60 Hz Power"=w144:bool, "Contactor Settings(*All Check Out).Station 5.50 Hz Power"=w145:bool, "Contactor Settings(*All Check Out).Station 5.120V Range"=w146:bool, "Contactor Settings(*All Check Out).Station 5.240V Range"=w147:bool, "Contactor Settings(*All Check Out).Station 5.Ground Line"=w148:bool, "Contactor Settings(*All Check Out).Station 5.Ground Neutral"=w149:bool, "Contactor Settings(*All Check Out).Station 5.Ground Leakage"=w133:T7, "Contactor Settings(*All Check Out).Station 5.Spare"=w132:bool, "Door Output Relays.Station 5 Freezer"=w150:bool, "Door Output Relays.Station 5 Cab"=w151:bool, "Door Output Relays.Station 5 Slide"=w152:bool)
      n47 = Boolean To (0,1)(Boolean=w144) -> (0, 1=w142:i16)
      n48 = Boolean To (0,1)(Boolean=w145) -> (0, 1=w141:i16)
      n49 = Boolean To (0,1)(Boolean=w146) -> (0, 1=w140:i16)
      n50 = Boolean To (0,1)(Boolean=w147) -> (0, 1=w139:i16)
      n51 = Boolean To (0,1)(Boolean=w148) -> (0, 1=w138:i16)
      n52 = Boolean To (0,1)(Boolean=w149) -> (0, 1=w137:i16)
      n53 = Boolean To (0,1)(Boolean=w132) -> (0, 1=w131:i16)
      n54 = Boolean To (0,1)(Boolean=w150) -> (0, 1=w136:i16)
      n55 = Boolean To (0,1)(Boolean=w151) -> (0, 1=w135:i16)
      n56 = Boolean To (0,1)(Boolean=w152) -> (0, 1=w134:i16)
    }
    frame 6 {
      n57 = Unbundle By Name(w177) -> ("Measured Input Data (Target).Voltage Setpoint 6 (*Volt Set6)"=w167:dbl, "Contactor Settings(*All Check Out).Station 6.60 Hz Power"=w168:bool, "Contactor Settings(*All Check Out).Station 6.50 Hz Power"=w169:bool, "Contactor Settings(*All Check Out).Station 6.120V Range"=w170:bool, "Contactor Settings(*All Check Out).Station 6.240V Range"=w171:bool, "Contactor Settings(*All Check Out).Station 6.Ground Line"=w172:bool, "Contactor Settings(*All Check Out).Station 6.Ground Neutral"=w173:bool, "Contactor Settings(*All Check Out).Station 6.Ground Leakage"=w157:T7, "Contactor Settings(*All Check Out).Station 6.Room Pump"=w156:bool, "Door Output Relays.Station 6 Freezer"=w174:bool, "Door Output Relays.Station 6 Cab"=w175:bool, "Door Output Relays.Station 6 Slide"=w176:bool)
      n58 = Boolean To (0,1)(Boolean=w168) -> (0, 1=w158:i16)
      n59 = Boolean To (0,1)(Boolean=w169) -> (0, 1=w159:i16)
      n60 = Boolean To (0,1)(Boolean=w170) -> (0, 1=w160:i16)
      n61 = Boolean To (0,1)(Boolean=w171) -> (0, 1=w161:i16)
      n62 = Boolean To (0,1)(Boolean=w172) -> (0, 1=w162:i16)
      n63 = Boolean To (0,1)(Boolean=w173) -> (0, 1=w163:i16)
      n64 = Boolean To (0,1)(Boolean=w156) -> (0, 1=w155:i16)
      n65 = Boolean To (0,1)(Boolean=w174) -> (0, 1=w164:i16)
      n66 = Boolean To (0,1)(Boolean=w175) -> (0, 1=w165:i16)
      n67 = Boolean To (0,1)(Boolean=w176) -> (0, 1=w166:i16)
    }
    frame 7 {
      n68 = Unbundle By Name(w201) -> ("Measured Input Data (Target).Voltage Setpoint 7 (*Volt Set7)"=w191:dbl, "Contactor Settings(*All Check Out).Station 7.60 Hz Power"=w192:bool, "Contactor Settings(*All Check Out).Station 7.50 Hz Power"=w193:bool, "Contactor Settings(*All Check Out).Station 7.120V Range"=w194:bool, "Contactor Settings(*All Check Out).Station 7.240V Range"=w195:bool, "Contactor Settings(*All Check Out).Station 7.Ground Line"=w196:bool, "Contactor Settings(*All Check Out).Station 7.Ground Neutral"=w197:bool, "Contactor Settings(*All Check Out).Station 7.Ground Leakage"=w181:T7, "Contactor Settings(*All Check Out).Station 7.Spare"=w180:bool, "Door Output Relays.Station 7 Freezer"=w198:bool, "Door Output Relays.Station 7 Cab"=w199:bool, "Door Output Relays.Station 7 Slide"=w200:bool)
      n69 = Boolean To (0,1)(Boolean=w192) -> (0, 1=w190:i16)
      n70 = Boolean To (0,1)(Boolean=w193) -> (0, 1=w189:i16)
      n71 = Boolean To (0,1)(Boolean=w194) -> (0, 1=w188:i16)
      n72 = Boolean To (0,1)(Boolean=w195) -> (0, 1=w187:i16)
      n73 = Boolean To (0,1)(Boolean=w196) -> (0, 1=w186:i16)
      n74 = Boolean To (0,1)(Boolean=w197) -> (0, 1=w185:i16)
      n75 = Boolean To (0,1)(Boolean=w180) -> (0, 1=w179:i16)
      n76 = Boolean To (0,1)(Boolean=w198) -> (0, 1=w184:i16)
      n77 = Boolean To (0,1)(Boolean=w199) -> (0, 1=w183:i16)
      n78 = Boolean To (0,1)(Boolean=w200) -> (0, 1=w182:i16)
    }
    frame 8 {
      n79 = Unbundle By Name(w225) -> ("Measured Input Data (Target).Voltage Setpoint 8 (*Volt Set8)"=w215:dbl, "Contactor Settings(*All Check Out).Station 8.60 Hz Power"=w216:bool, "Contactor Settings(*All Check Out).Station 8.50 Hz Power"=w217:bool, "Contactor Settings(*All Check Out).Station 8.120V Range"=w218:bool, "Contactor Settings(*All Check Out).Station 8.240V Range"=w219:bool, "Contactor Settings(*All Check Out).Station 8.Ground Line"=w220:bool, "Contactor Settings(*All Check Out).Station 8.Ground Neutral"=w221:bool, "Contactor Settings(*All Check Out).Station 8.Ground Leakage"=w205:T7, "Contactor Settings(*All Check Out).Station 8.Spare"=w204:bool, "Door Output Relays.Station 8 Freezer"=w222:bool, "Door Output Relays.Station 8 Cab"=w223:bool, "Door Output Relays.Station 8 Slide"=w224:bool)
      n80 = Boolean To (0,1)(Boolean=w216) -> (0, 1=w214:i16)
      n81 = Boolean To (0,1)(Boolean=w217) -> (0, 1=w213:i16)
      n82 = Boolean To (0,1)(Boolean=w218) -> (0, 1=w212:i16)
      n83 = Boolean To (0,1)(Boolean=w219) -> (0, 1=w211:i16)
      n84 = Boolean To (0,1)(Boolean=w220) -> (0, 1=w210:i16)
      n85 = Boolean To (0,1)(Boolean=w221) -> (0, 1=w209:i16)
      n86 = Boolean To (0,1)(Boolean=w204) -> (0, 1=w203:i16)
      n87 = Boolean To (0,1)(Boolean=w222) -> (0, 1=w208:i16)
      n88 = Boolean To (0,1)(Boolean=w223) -> (0, 1=w207:i16)
      n89 = Boolean To (0,1)(Boolean=w224) -> (0, 1=w206:i16)
    }
  }
  n90 = Build Array(w6) -> (w23:dbl[])
  n91 = Build Array(w7) -> (w24:i16[])
  n92 = Build Array(w8) -> (w25:i16[])
  n93 = Build Array(w9) -> (w26:i16[])
  n94 = Build Array(w10) -> (w27:i16[])
  n95 = Build Array(w11) -> (w28:i16[])
  n96 = Build Array(w12) -> (w29:i16[])
  n97 = Build Array(w13) -> (w30:T7[])
  n98 = Build Array(w14) -> (w31:i16[])
  n99 = Build Array(w15) -> (w32:i16[])
  n100 = Build Array(w16) -> (w33:i16[])
  n101 = Build Array(w17) -> (w34:i16[])
  n102 = Build Array(w23, w24, w25, w26, w27, w28, w29, w30, w31, w32, w33, w34) -> (w20:dbl[][])
  n103 = Index Array(array=w20, index (col)=0 ("disabled index (col)")) -> (element=w18:dbl[])  [unwired: 1 in]
  "Data 4 (DBL)" <- w18
  n104 = call "UTILITY Double Array to String Array.vi"("Hex Array Out"=w18) -> ("Array"=w21:string[])  [unwired: 10 in]
  n105 = Build Array(w22, w21) -> (w2:string[][])
  n106 = Transpose 2D Array(2D array=w2) -> (transposed array=→"Data 4":string[][])
  "Error Out" <- "Error In"
  "Chamber 1 Data Out" <- "Chamber 1 Data in"
